vi "Parse Identity from Result.vi"(8 "error in (no error)":errorcluster, 11 "ReadCommand In":refnum<class "ReadCommand.lvclass">) -> (0 "error out":errorcluster, 3 "Identity":string)   [LabVIEW 2023]
doc: "Obtains the result from the Read Command and returns it as the Instrument Identity. Raw Result, from Read Command, is actually a String so is already in a useable format; other values can be obtained from that Raw Result by using helper VIs in Virtual Folder Data Types."
uses:
  IDN/IDN.lvclass
  ReadCommand/ReadCommand.lvclass
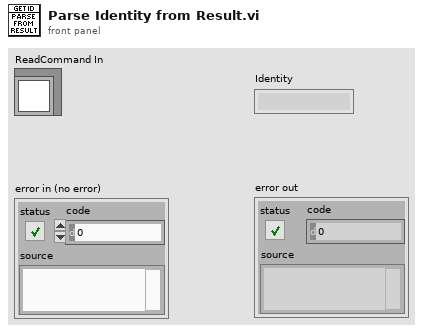
[diagram p1: front panel]
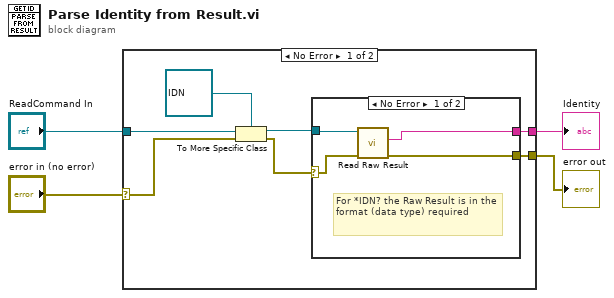
[diagram p0: block diagram]
diagram:
  n1 = case shown="No Error" "error in (no error)" {
    selector: "error in (no error)" -> [w10 w17]
    tunnel: "ReadCommand In" -> [w11 _]
    tunnel: [w6 _] -> w2
    tunnel: [w5 w17] -> w1
    frame No Error {
      n2 = To More Specific Class(target class=refnum<class "IDN.lvclass"> refnum ("HAF:IDN.lvclass"), reference=w11, error in=w10) -> (specific class reference=w7:refnum<class "IDN.lvclass">, error out=w8:errorcluster)
      n3 = case shown="No Error" w8 {
        selector: w8 -> [w14 w16]
        tunnel: w7 -> [w15 _]
        tunnel: [w13 _] -> w6
        tunnel: [w12 w16] -> w5
        frame No Error {
          # "For *IDN? the Raw Result is in the format (data type) required"
          n4 = call-dynamic "Read Raw Result.vi"("error in (no error)"=w14, "ReadCommand in"=w15) -> ("error out"=w12:errorcluster, "Raw Result"=w13:string)  [unwired: 7 in, 1 out]
        }
        frame Error {
        }
      }
    }
    frame Error {
    }
  }
  "error out" <- w1
  "Identity" <- w2
